vi "divide.vi"(8 "error in (no error)":errorcluster, 9 "divisor":dbl=1.0, 10 "divisor":refnum<class "ImageCollection.lvclass">, 11 "ImageCollection in":refnum<class "ImageCollection.lvclass">) -> (0 "error out":errorcluster, 3 "ImageCollection out":refnum<class "ImageCollection.lvclass">)   [LabVIEW 2010, in "ImageCollection.lvclass"]
uses:
  ImageCollection.lvclass
  Image/Image/Image.lvclass
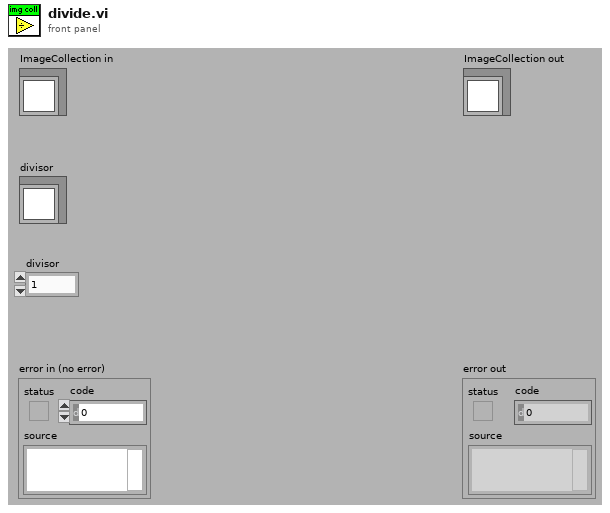
[diagram p1: front panel]
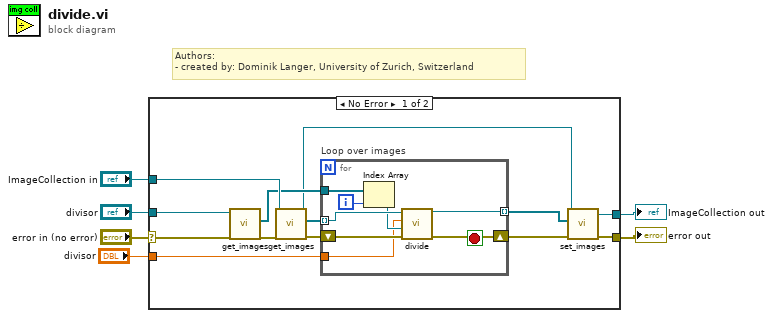
[diagram p0: block diagram]
diagram:
  # "Authors: \n- created by: Dominik Langer, University of Zurich, Switzerland"
  n1 = case shown="No Error" "error in (no error)" {
    selector: "error in (no error)" -> [w19 w29]
    tunnel: [w12 w29] -> w5
    tunnel: [w9 w28] -> w3
    tunnel: "ImageCollection in" -> [w17 w28]
    tunnel: "divisor" -> [w8 _]
    tunnel: "divisor" -> [w7 _]
    frame No Error {
      n2 = call-dynamic "get_images.vi"("error in (no error)"=w19, "ImageCollection.lvclass in"=w8) -> ("error out"=w18:errorcluster, "images"=w14:refnum<class "Image.lvclass">[])  [unwired: 8 out]
      n3 = call-dynamic "get_images.vi"("error in (no error)"=w18, "ImageCollection.lvclass in"=w17) -> ("error out"=w16:errorcluster, "images"=w15:refnum<class "Image.lvclass">[], "ImageCollection.lvclass out"=w10:refnum<class "ImageCollection.lvclass">)  [unwired: 7 out]
      n4 = for "Loop over images" {
        shift-right: [w20] -> w13
        shift-left: w16 -> [w27]
        tunnel: w15 -> [w25] mode=indexing
        tunnel: w14 -> [w24]
        tunnel: [w26] -> w11 mode=indexing
        tunnel: w7 -> [w21]
        i -> [w23]
        stop <- w20 stop-if-true
        n5 = Index Array(array=w24, index=w23) -> (element=w22:refnum<class "Image.lvclass">)
        n6 = call-dynamic "divide.vi"("error in (no error)"=w27, 9:"divisor"=w22, 10:"divisor"=w21, "Image in"=w25) -> ("error out"=w20:errorcluster, "Image out"=w26:refnum<class "Image.lvclass">)  [unwired: 6 out]
      }
      n7 = call-dynamic "set_images.vi"("error in (no error)"=w13, "images"=w11, "ImageCollection.lvclass in"=w10) -> ("error out"=w12:errorcluster, "ImageCollection.lvclass out"=w9:refnum<class "ImageCollection.lvclass">)  [unwired: 7 out]
    }
    frame Error {
    }
  }
  "error out" <- w5
  "ImageCollection out" <- w3
